vi "Init.vi"(8 "error in (no error)":errorcluster, 9 "SA Pin":string, 10 "Measurement Name":string) -> (0 "error out":errorcluster, 3 "WCDMA ACP out":refnum<class "WCDMA ACP.lvclass">)   [LabVIEW 2016, in "SeqAuto Evaluations.lvlib" / "WCDMA ACP.lvclass"]
uses:
  WCDMA ACP.lvclass
  C:/Sequence Automation/Plugins/SeqAuto IEvaluation.lvlibp/SeqAuto IEvaluation.lvclass
  WCDMA ACP.lvclass/WCDMA ACP.ctl
  Plugins/SeqAuto IEvaluation.lvlibp/Write Measurement Name.vi
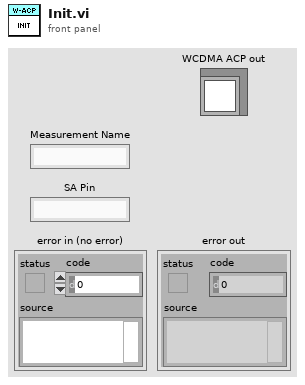
[diagram p1: front panel]
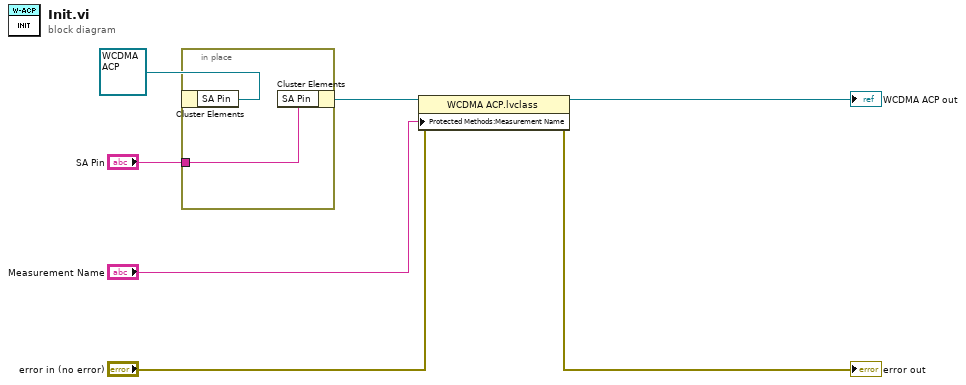
[diagram p0: block diagram]
diagram:
  n1 = in-place {
    in-place-border: "SA Pin" -> [w8]
    n2 = in-place-cluster #1(refnum<class "WCDMA ACP.lvclass"> refnum ("WCDMA ACP in")) -> ()  [unwired: 1 out]
    n3 = in-place-cluster #1("SA Pin"=w8) -> (w3:refnum<class "WCDMA ACP.lvclass">)
  }
  n4 = property class="WCDMA ACP.lvclass"(reference=w3, error in="error in (no error)", "Protected Methods:Measurement Name"="Measurement Name") -> (reference out=→"WCDMA ACP out":refnum<class "WCDMA ACP.lvclass">, error out=→"error out":errorcluster)
